vi "biexp levenberg.vi"(5 "derivative":T1(ring), 6 "Standard Deviation":dbl[](array[numeric]) format="%.2f", 7 "max iteration":i32=200, 8 "Initial Guess Coefficients":dbl[](array[numeric]) format="%.2f", 9 "Y":dbl[](array[numeric]) format="%.2f", 10 "X":dbl[](array[numeric]) format="%.2f") -> (0 "error":i32, 1 "mse":dbl format="%.4e", 2 "Best Fit":dbl[](array[numeric]) format="%.2f", 3 "Best Fit Coefficients":dbl[](array[numeric]) format="%.2f", 4 "Covariance":dbl[][](array[numeric]) format="%.2f")   [LabVIEW 2009]
uses:
  <vilib>/Analysis/baseanly.llb/Real Inverse Matrix.vi
  <vilib>/Analysis/NI_AALBase.lvlib
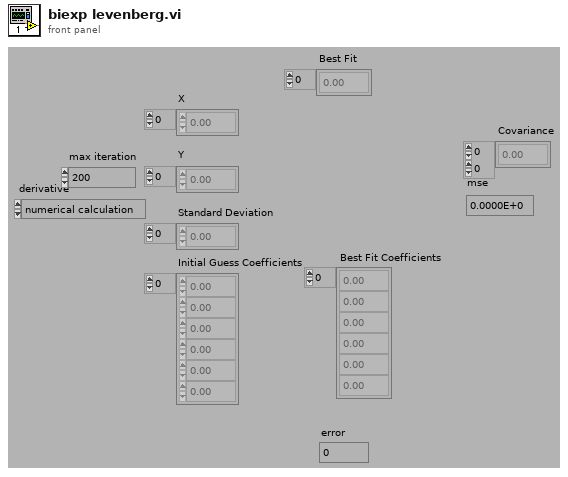
[diagram p1: front panel]
types:
  T1 = enum32{"numerical calculation", "formula calculation"}
  T2 = typedef "NI_Matrix.lvlib/RealMatrix.ctl" = dbl[][]
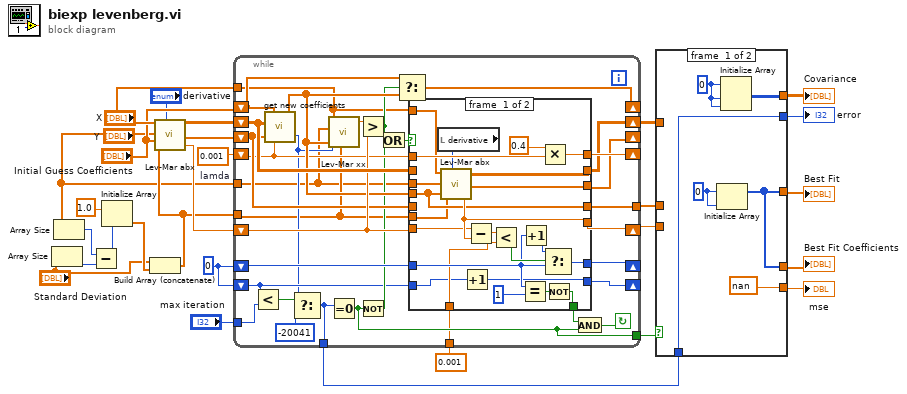
[diagram p0: block diagram]
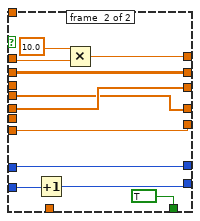
[diagram p2: hidden frame]
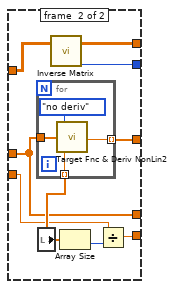
[diagram p3: hidden frame]
diagram:
  w17 = 0
  w26 = 0.001  # lamda
  n1 = Array Size(array="Standard Deviation") -> (size(s)=w6:i32)
  n2 = Array Size(array="Y") -> (size(s)=w7:i32)
  n3 = Subtract(x=w7, y=w6) -> (x-y=w5:i32)
  n4 = Initialize Array(1.0, w5) -> (w4:dbl[])
  n5 = Build Array (concatenate)("Standard Deviation", w4) -> (w2:dbl[])
  n6 = call "Lev-Mar abx.vi"("X"="X", "Y"="Y", "Coefficients"="Initial Guess Coefficients", "Standard Deviation"=w2, "derivative"="derivative") -> ("Alpha"=w27:dbl[][], "Beta"=w25:dbl[], "chiSqr"=w24:dbl)
  n7 = while {
    tunnel: "X" -> [w29]
    tunnel: "Y" -> [w31]
    tunnel: [w32] -> w9
    tunnel: "max iteration" -> [w34]
    tunnel: w2 -> [w33]
    shift-left: w17 -> [w38]
    shift-right: [w39] -> _
    tunnel: 0.001 -> [w43]
    tunnel: [w44] -> w19
    tunnel: [w47] -> w22
    shift-left: w17 -> [w52]
    shift-right: [w51] -> _
    shift-left: w24 -> [w53]
    shift-right: [w54] -> w23
    shift-left: w25 -> [w50]
    shift-right: [w55] -> _
    shift-left: w27 -> [w56]
    shift-right: [w57] -> w8
    shift-left: "Initial Guess Coefficients" -> [w30]
    shift-right: [w58] -> _
    shift-left: w26 -> [w48]
    shift-right: [w59] -> _
    stop <- w46 continue-if-true
    n8 = Less?(x=w38, y=w34) -> (x < y?=w37:bool)
    n9 = call "get new coefficients.vi"("lamda"=w48, "Beta"=w50, "Alpha"=w56, "Coefficients"=w30) -> ("error"=w35:i32, "New Coefficients"=w49:dbl[])
    n10 = Select(t=w35, s=w37, f=-20041) -> (s? t:f=w32:i32)
    n11 = call "Lev-Mar xx.vi"("X"=w29, "Y"=w31, "Coefficients"=w49, "error"=w35, "Standard Deviation"=w33) -> ("chiSqr"=w60:dbl)
    n12 = Equal To 0?(x=w32) -> (x = 0?=w44:bool)
    n13 = Greater?(x=w60, y=w53) -> (0:w41:bool)
    n14 = Not(x=w44) -> (.not. x?=w40:bool)
    n15 = Or(x=w41, y=w40) -> (x .or. y?=w42:bool)
    n16 = Select(t=w30, s=w41, f=w49) -> (s? t:f=w58:dbl[])
    n17 = case shown="False" w42 {
      tunnel: w48 -> [w82 w93]
      tunnel: [w81 w92] -> w59
      tunnel: [w80 w91] -> w57
      tunnel: w56 -> [_ w91]
      tunnel: [w79 w87] -> w55
      tunnel: [w78 w90] -> w54
      tunnel: w53 -> [w77 w90]
      tunnel: w52 -> [w72 w89]
      tunnel: [w73 w89] -> w51
      tunnel: [w69 TRUE] -> w45
      tunnel: w49 -> [w66 w86]
      tunnel: w50 -> [_ w87]
      tunnel: [w66 w86] -> w47
      tunnel: w43 -> [w68 _]
      tunnel: [w63 w85] -> w39
      tunnel: w38 -> [w67 w84]
      tunnel: w33 -> [w65 _]
      tunnel: w29 -> [w62 _]
      tunnel: w31 -> [w61 _]
      frame #0 {
        n18 = local read "derivative"() -> (w64:T1)
        n19 = call "Lev-Mar abx.vi"("X"=w62, "Y"=w61, "Coefficients"=w66, "Standard Deviation"=w65, "derivative"=w64) -> ("Alpha"=w80:dbl[][], "Beta"=w79:dbl[], "chiSqr"=w78:dbl)
        n20 = Increment(x=w67) -> (x+1=w63:i32)
        n21 = Subtract(x=w77, y=w78) -> (x-y=w76:dbl)
        n22 = Less?(x=w76, y=w68) -> (x < y?=w75:bool)
        n23 = Equal?(x=w72, y=1) -> (x = y?=w70:bool)
        n24 = Increment(x=w72) -> (x+1=w74:i32)
        n25 = Multiply(x=0.4, y=w82) -> (x*y=w81:dbl)
        n26 = Select(t=w74, s=w75, f=w72) -> (s? t:f=w73:i32)
        n27 = Not(x=w70) -> (.not. x?=w69:bool)
      }
      frame #1 {
        n28 = Increment(x=w84) -> (x+1=w85:i32)
        n29 = Multiply(x=10.0, y=w93) -> (x*y=w92:dbl)
      }
    }
    n30 = And(x=w45, y=w44) -> (x .and. y?=w46:bool)
  }
  n31 = case shown="True" w19 {
    tunnel: w22 -> [_ w105]
    tunnel: [w98 w105] -> w21
    tunnel: [nan w109] -> w20
    tunnel: [w98 w106] -> w12
    tunnel: w23 -> [_ w104]
    tunnel: [w96 w103] -> w11
    tunnel: [w95 w102] -> w10
    tunnel: w9 -> [w95 _]
    tunnel: w8 -> [_ w101]
    frame #0 {
      w97 = 0
      w100 = 0
      n32 = Initialize Array(w100, w100) -> (w98:i32[])
      n33 = Initialize Array(w97, w97, w97) -> (w96:i32[][])
    }
    frame #1 {
      n34 = local read "X"() -> (w108:dbl[])
      n35 = for {
        tunnel: w105 -> [w112]
        tunnel: [w111] -> w106 mode=indexing
        tunnel: w108 -> [w113] mode=indexing
        n36 = call "Target Fnc & Deriv NonLin2.vi"("X"=w113, "Coefficients"=w112, "Flag"=enum16{"no deriv", "deriv"}."no deriv") -> ("Y"=w111:dbl)  [unwired: 1 out]
      }
      n37 = call-poly <vilib>:"Inverse Matrix.vi"("Input Matrix"=w101) -> ("error"=w102:i32, "Inverse Matrix"=w103:T2)  [unwired: 1 in]
      n38 = Array Size(array=w108) -> (size(s)=w107:i32)
      n39 = Divide(x=w104, y=w107) -> (x/y=w109:dbl)
    }
  }
  "mse" <- w20
  "Best Fit Coefficients" <- w21
  "Best Fit" <- w12
  "error" <- w10
  "Covariance" <- w11
